vi "test_CCDGetDataSize.vi"(6 "Delay between send and receive [ms]":i32=100, 7 "Test should pass":bool=TRUE, 8 "error in":errorcluster, 9 "tear down connection":bool=TRUE, 10 "set-up a connection":bool=TRUE, 11 "device selection":enum16{"monochromator", "CCD", "SCD"}(ring)=enum."CCD") -> (0 "error out":errorcluster)   [LabVIEW 2023]
uses:
  Classes/CCD/CCD.lvclass
  <vilib>/addons/_JKI Toolkits/Caraya/classes/Assert/Assert Not Error.vi
  <vilib>/addons/_JKI Toolkits/Caraya/classes/Assert/Assert Equal Value and Type_Variant.vi
  <vilib>/addons/_JKI Toolkits/Caraya/classes/Test/Test.lvclass
  <vilib>/addons/_JKI Toolkits/Caraya/classes/Assert/Assert.lvclass
panel:
  # "Connector Pane"
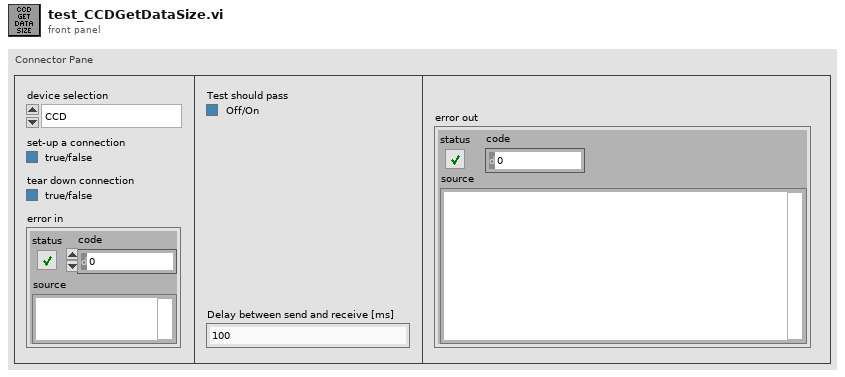
[diagram p1: front panel]
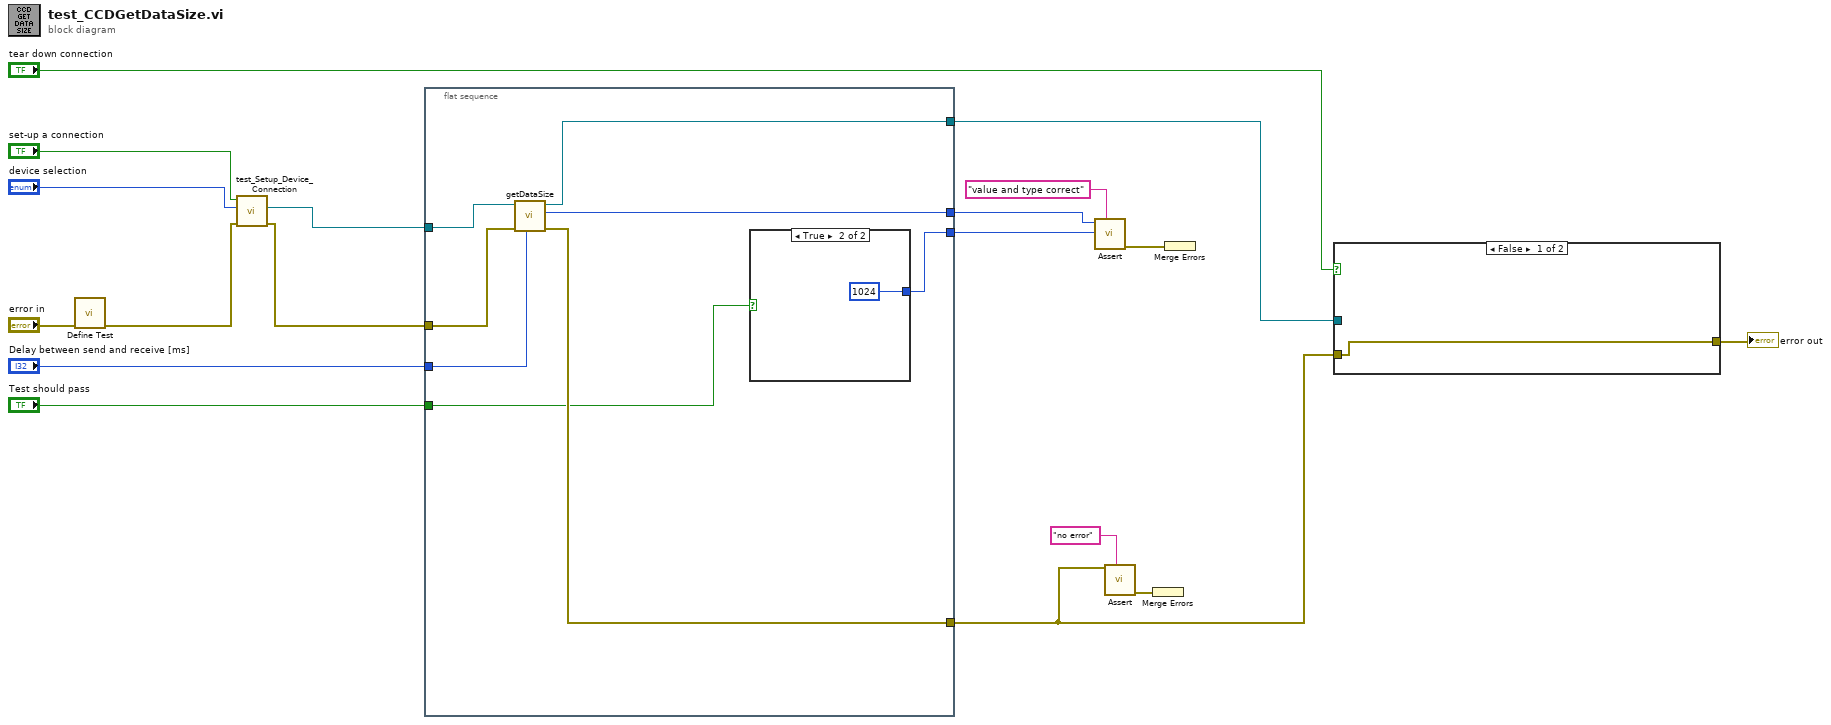
[diagram p0: block diagram]
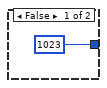
[diagram p2: hidden frame]
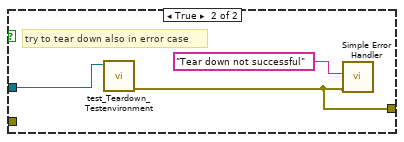
[diagram p3: hidden frame]
diagram:
  n1 = call <vilib>:"Define Test.vi"("error in (no error)"="error in") -> ("error out"=w2:errorcluster)  [unwired: 9 in, 1 out]
  n2 = call "test_Setup_Device_Connection.vi"("error in (no error)"=w2, "device selection"="device selection", "set-up a connection"="set-up a connection") -> ("error out"=w3:errorcluster, "CCD.lvclass"=w4:refnum<class "CCD.lvclass">)  [unwired: 5 in, 2 out]
  n3 = flat-sequence {
    tunnel: [w23] -> w16
    tunnel: w3 -> [w26]
    tunnel: w4 -> [w25]
    tunnel: [w22] -> w14
    tunnel: [w24] -> w9
    tunnel: "Test should pass" -> [w21]
    tunnel: [w20] -> w8
    tunnel: "Delay between send and receive [ms]" -> [w19]
    frame #0 {
      n4 = call "getDataSize.vi"("Delay between send and receive [ms]"=w19, "error in (no error)"=w26, "CCD in"=w25) -> ("error out"=w24:errorcluster, "size"=w23:i32, "CCD out"=w20:refnum<class "CCD.lvclass">)  [unwired: 6 in]
      n5 = case shown="True" w21 {
        tunnel: [1023 1024] -> w22
        frame False {
        }
        frame True {
        }
      }
    }
  }
  n6 = call-poly <vilib>:"Assert.vi"("Label"="value and type correct" ("Label (VI Title)"), "Y"=w14, "X"=w16) -> ("error out"=w17:errorcluster)  [unwired: 7 in, 1 out]
  n7 = call-poly <vilib>:"Assert.vi"("Label"="no error" ("Label (VI Title)"), "Not Error?"=w9) -> ("error out"=w11:errorcluster)  [unwired: 8 in, 1 out]
  n8 = Merge Errors(w11) -> ()  [unwired: 1 out]
  n9 = Merge Errors(w17) -> ()  [unwired: 1 out]
  n10 = case shown="False" "tear down connection" {
    tunnel: w8 -> [_ w31]
    tunnel: [w29 w30] -> w7
    tunnel: w9 -> [w29 _]
    frame False {
    }
    frame True {
      # "try to tear down also in error case"
      n11 = call "test_Teardown_Testenvironment.vi"("GenericDevice.lvclass"=w31) -> ("error out"=w30:errorcluster)  [unwired: 9 in, 1 out]
      n12 = call <vilib>:"Simple Error Handler.vi"("error source (\" \")"="Tear down not successful" ("error source (\" \")"), "error in (no error)"=w30) -> ()  [unwired: 3 in, 5 out]
    }
  }
  "error out" <- w7
